vi "Point-in-Tri test (barycentric coords).vi"(1 "Point":sgl[](array[numeric]), 2 "Triangle":T1) -> (0 "Point is inside triangle":bool)   [LabVIEW 2014]
uses:
  Typedefs/Triangle.ctl
panel:
  # "PN 13/01/2015"
  # "Vertices"
  # "Edges"
  # "Unit normal"
  # "pre-store"
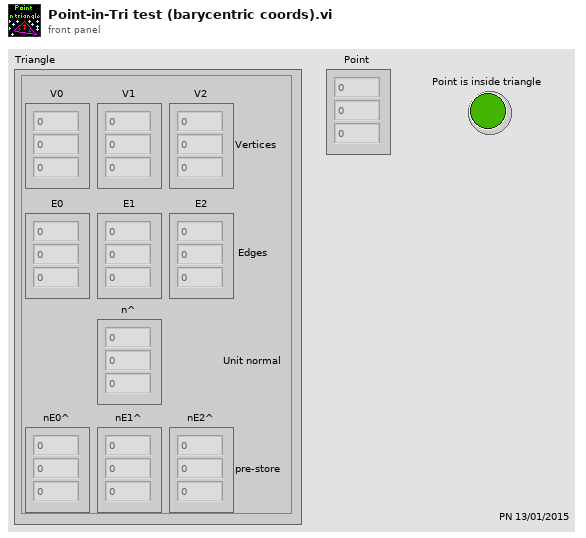
[diagram p1: front panel]
types:
  T1 = typedef "Triangle.ctl" = cluster{"V0":sgl[], "V1":sgl[], "V2":sgl[], "E0":sgl[], "E1":sgl[], "E2":sgl[], "n^":sgl[], "nE0^":sgl[], "nE1^":sgl[], "nE2^":sgl[]}
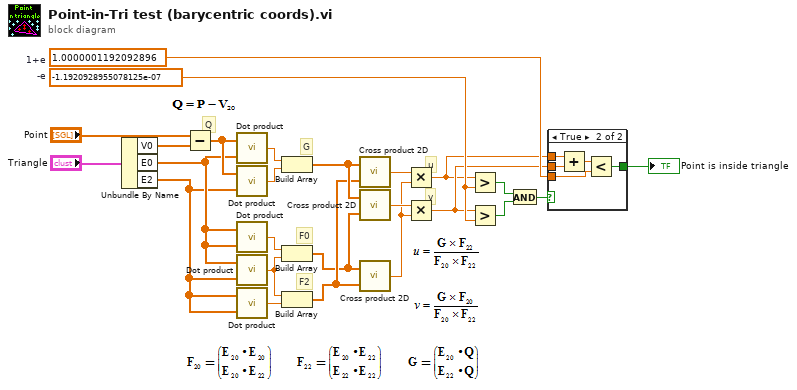
[diagram p0: block diagram]
diagram:
  w16 = sgl -1.1920929e-07  # -e
  w12 = sgl 1.0000001  # 1+e
  # "F2"
  # "F0"
  # "v"
  # "u"
  # "G"
  # "Q"
  n1 = Unbundle By Name("Triangle") -> ("V0"=w23:sgl[], "E0"=w8:sgl[], "E2"=w6:sgl[])
  n2 = Subtract(x="Point", y=w23) -> (x-y=w22:sgl[])
  n3 = call "Dot product.vi"("B"=w8, "A"=w22) -> ("A . B"=w21:sgl)
  n4 = call "Dot product.vi"("B"=w6, "A"=w22) -> ("A . B"=w20:sgl)
  n5 = call "Dot product.vi"("B"=w8, "A"=w8) -> ("A . B"=w7:sgl)
  n6 = call "Dot product.vi"("B"=w6, "A"=w8) -> ("A . B"=w5:sgl)
  n7 = call "Dot product.vi"("B"=w6, "A"=w6) -> ("A . B"=w4:sgl)
  n8 = Build Array(w21, w20) -> (w18:sgl[])
  n9 = Build Array(w7, w5) -> (w1:sgl[])
  n10 = Build Array(w5, w4) -> (w2:sgl[])
  n11 = call "Cross product 2D.vi"("B"=w2, "A"=w18) -> ("A X B"=w19:sgl)
  n12 = call "Cross product 2D.vi"("B"=w1, "A"=w18) -> ("A X B"=w17:sgl)
  n13 = call "Cross product 2D.vi"("B"=w2, "A"=w1) -> ("A X B"=w3:sgl)
  n14 = Multiply(x=w19, y=w3) -> (x*y=w10:sgl)
  n15 = Multiply(x=w17, y=w3) -> (x*y=w11:sgl)
  n16 = Greater?(x=w10, y=w16) -> (0:w15:bool)
  n17 = Greater?(x=w11, y=w16) -> (0:w14:bool)
  n18 = And(x=w15, y=w14) -> (x .and. y?=w13:bool)
  n19 = case shown="True" w13 {
    selector: w13 -> [w26 _]
    tunnel: w10 -> [_ w31]
    tunnel: w11 -> [_ w30]
    tunnel: w12 -> [_ w28]
    tunnel: [w26 w27] -> w9
    frame False {
    }
    frame True {
      n20 = Add(x=w31, y=w30) -> (x+y=w29:sgl)
      n21 = Less?(x=w29, y=w28) -> (x < y?=w27:bool)
    }
  }
  "Point is inside triangle" <- w9
